vi "SetValueByItemName.vi"(0 "VI Reference In":refnum<vi>, 2 "delimiter (>>)":string=">>", 5 "Control Path":string, 7 "Item Name":string, 9 "Occurance":i32=1, 11 "Error In":errorcluster) -> (4 "VI Reference Out":refnum<vi>, 15 "Error Out":errorcluster)   [LabVIEW 2016, in "Drona.lvlib" / "ControlValue.lvlib"]
doc: "Sets value(signaling) for the listbox control whose item name is specified. \n\nThe input control name is given as a string , incase of path, use delimiters inbetween the path."
uses:
  ControlValue.lvlib
  <vilib>/Utility/error.llb/Error Cluster From Error Code.vi
  <vilib>/ErrorRing/Error Ring.xnode
  Drona.lvlib
  Get/GetControlRef/GetControlRef.lvlib
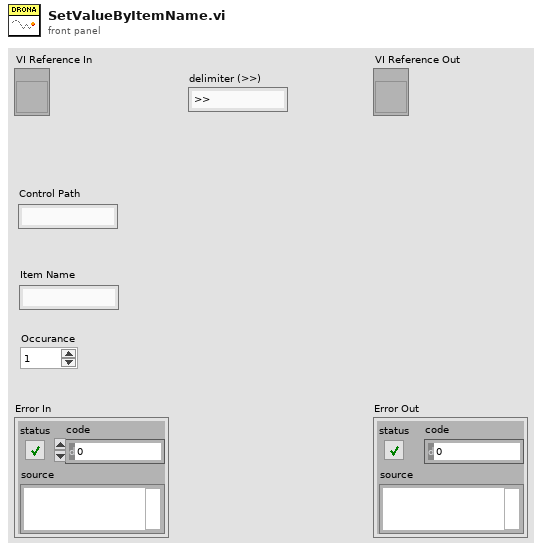
[diagram p1: front panel]
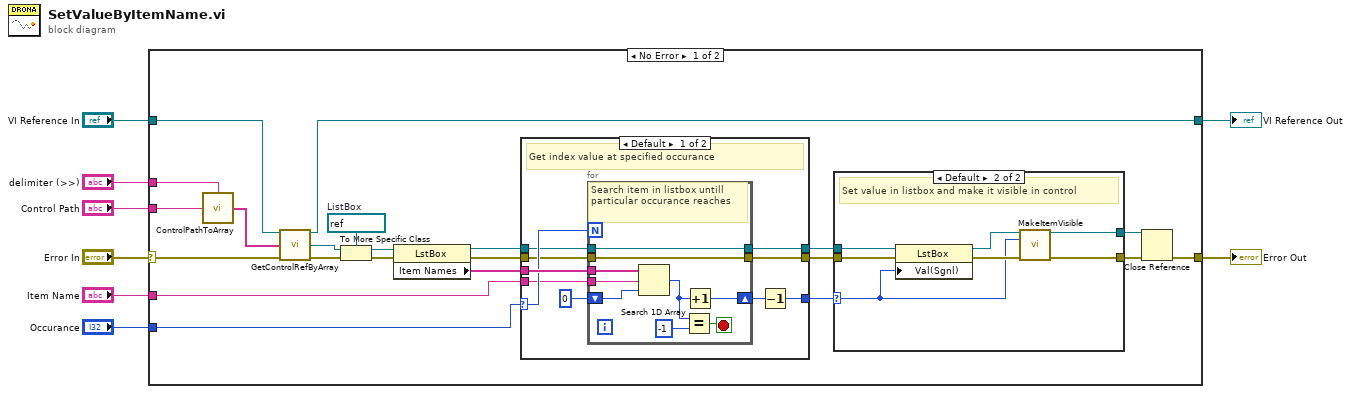
[diagram p0: block diagram]
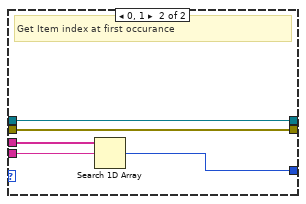
[diagram p2: hidden frame]
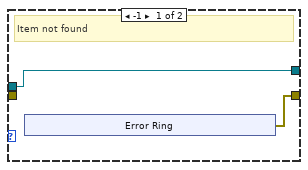
[diagram p3: hidden frame]
diagram:
  n1 = case shown="No Error" "Error In" {
    selector: "Error In" -> [w24 w70]
    tunnel: [w25 w70] -> w7
    tunnel: "VI Reference In" -> [w23 w69]
    tunnel: "Control Path" -> [w27 _]
    tunnel: [w12 w69] -> w4
    tunnel: "delimiter (>>)" -> [w26 _]
    tunnel: "Item Name" -> [w18 _]
    tunnel: "Occurance" -> [w17 _]
    frame No Error {
      w29 = refnum<vi> refnum  # ListBox
      n2 = call "ControlPathToArray.vi"("Control Name"=w27, "delimiter (>>)"=w26) -> ("Control Path"=w22:string[])
      n3 = call "GetControlRefByArray.vi"("VI Reference In"=w23, "Control Path"=w22, "error In"=w24) -> ("VI Reference Out"=w12:refnum<vi>, "Ctl Refnum"=w20:refnum<vi>, "error out"=w21:errorcluster)  [unwired: 10 in]
      n4 = To More Specific Class(target class=w29, reference=w20, error in=w21) -> (specific class reference=w28:refnum<vi>, error out=w30:errorcluster)
      n5 = property class="LstBox"(reference=w28, error in=w30) -> (reference out=w14:refnum<vi>, error out=w16:errorcluster, "Item Names"=w19:string[])
      n6 = case shown="Default" w17 {
        selector: w17 -> [w39 _]
        tunnel: w19 -> [w40 w54]
        tunnel: w18 -> [w37 w53]
        tunnel: [w35 w52] -> w10
        tunnel: w16 -> [w34 w51]
        tunnel: [w33 w51] -> w15
        tunnel: w14 -> [w32 w50]
        tunnel: [w31 w50] -> w13
        frame Default {
          # "Get index value at specified occurance"
          n7 = for {
            N: w39 -> [_]
            tunnel: w40 -> [w49]
            tunnel: w37 -> [w47]
            shift-right: [w46] -> w36
            shift-left: 0 ("start index (0)") -> [w48]
            tunnel: w34 -> [w45]
            tunnel: [w45] -> w33
            tunnel: w32 -> [w44]
            tunnel: [w44] -> w31
            stop <- w43 stop-if-true
            # "Search item in listbox untill particular occurance reaches"
            n8 = Search 1D Array(1D array=w49, element=w47, start index (0)=w48) -> (index of element=w42:i32)
            n9 = Equal?(x=w42, y=-1) -> (x = y?=w43:bool)
            n10 = Increment(x=w42) -> (x+1=w46:i32)
          }
          n11 = Decrement(x=w36) -> (x-1=w35:i32)
        }
        frame 0, 1 {
          # "Get Item index at first occurance"
          n12 = Search 1D Array(1D array=w54, element=w53) -> (index of element=w52:i32)  [unwired: 1 in]
        }
      }
      n13 = case shown="Default" w10 {
        selector: w10 -> [_ w63]
        tunnel: w15 -> [_ w68]
        tunnel: w13 -> [w56 w67]
        tunnel: [w55 w65] -> w11
        tunnel: [w56 w62] -> w9
        frame -1 {
          # "Item not found"
          n14 = xnode "Error Ring"() -> ("error out"=w55:errorcluster)
        }
        frame Default {
          # "Set value in listbox and make it visible in control"
          n15 = property class="LstBox"(reference=w67, error in=w68, "Val(Sgnl)"=w63) -> (reference out=w64:refnum<vi>, error out=w66:errorcluster)
          n16 = call "MakeItemVisible.vi"("ListBox in"=w64, "Item Index"=w63, "error in (no error)"=w66) -> ("ListBox out"=w62:refnum<vi>, "error out"=w65:errorcluster)  [unwired: 11 in]
        }
      }
      n17 = Close Reference(reference=w9, error in (no error)=w11) -> (error out=w25:errorcluster)
    }
    frame Error {
    }
  }
  "Error Out" <- w7
  "VI Reference Out" <- w4
